vi "read_write_p.vi"() -> ()   [LabVIEW 2020]
uses:
  dxl_x86_c.lvlib/dxl_x86_c.lvlib
panel:
  out "dynamixel_comm_result":string
  out "dynamixel_error":string
  in  "Serial Port":string="COM1"
  in  "ADDR_PRESENT_POSITION":u16=580
  in  "ADDR_GOAL_POSITION":u16=564
  in  "ADDR_TORQUE_ENABLE":u16=512
  out "Protocol Version":dbl=2.0
  out "Present Position":i32(knob) scale=200000.0..-200000.0
  in  "terminate":bool
  out "port_num":i32
  in  "Goal Position":i32(knob) scale=200000.0..-200000.0
  in  "DYNAMIXEL ID":u8=1
  in  "Baud Rate":i32=57600
  # "/*******************************************************************************\n* Copyright (c) 2021, ROBOTIS CO., LTD.\n* All rights reserved.\n*\n* Redistribution and use in source and binary forms, with or without\n* modification, are permitted provided that the following conditions are met:\n*\n* * Redistributions of source code must retain the above copyright notice, this\n*   list of conditions and the following disclaimer.\n*\n* * Redistributions in binary form must reproduce the above copyright notice,\n*   this list of conditions and the following disclaimer in the documentation\n*   and/or other materials provided with the distribution.\n*\n* * Neither the name of ROBOTIS nor the names of its\n*   contributors may be used to endorse or promote products derived from\n*   this software without specific prior written permission.\n*\n* THIS SOFTWARE IS PROVIDED BY THE COPYRIGHT HOLDERS AND CONTRIBUTORS \"AS IS\"\n* AND ANY EXPRESS OR IMPLIED WARRANTIES, INCLUDING, BUT NOT LIMITED TO, THE\n* IMPLIED WARRANTIES OF MERCHANTABILITY AND FITNESS FOR A PARTICULAR PURPOSE ARE\n* DISCLAIMED. IN NO EVENT SHALL THE COPYRIGHT HOLDER OR CONTRIBUTORS BE LIABLE\n* FOR ANY DIRECT, INDIRECT, INCIDENTAL, SPECIAL, EXEMPLARY, OR CONSEQUENTIAL\n* DAMAGES (INCLUDING, BUT NOT LIMITED TO, PROCUREMENT OF SUBSTITUTE GOODS OR\n* SERVICES; LOSS OF USE, DATA, OR PROFITS; OR BUSINESS INTERRUPTION) HOWEVER\n* CAUSED AND ON ANY THEORY OF LIABILITY, WHETHER IN CONTRACT, STRICT LIABILITY,\n* OR TORT (INCLUDING NEGLIGENCE OR OTHERWISE) ARISING IN ANY WAY OUT OF THE USE\n* OF THIS SOFTWARE, EVEN IF ADVISED OF THE POSSIBILITY OF SUCH DAMAGE.\n*******************************************************************************/\n\n/* Author: Ryu Woon Jung (Leon), Will Son */"
  # "[How to run the example]\n1. Connect the U2D2 and DYNAMIXEL to the PC\n2. Confirm the Serial Port number that is assigned to the U2D2 from the Device Manager.\n3. Click the \"Run\" button to run the example.\n4. Drag the Goal Position dial knob or enter the value in the textbox underneath\n5. To finish the example, press \"Quit\" button. (Quitting with \"Abort Execution\" may cause port issue)\n\nSupported DYNAMIXEL with this example :\n  - All P series\n  - PRO(A) series : PRO series with Advanced firmware\n  - PRO series requires modification in ADDR_* fields\n\nThis example is designed for running DYNAMIXEL with U2D2.\nOther DYNAMIXEL such as X or PRO series can be run by modifying below address based on eManual.\nhttps://emanual.robotis.com\n  - ADDR_TORQUE_ENABLE\n  - ADDR_GOAL_POSITION\n  - ADDR_PRESENT_POSITION\n\nMake sure that your DYNAMIXEL is set to ID = 1, Baud Rate = 57600\nThese are the factory default setting of P series\n\nPlease note each P series have different MIN / MAX Position limits."
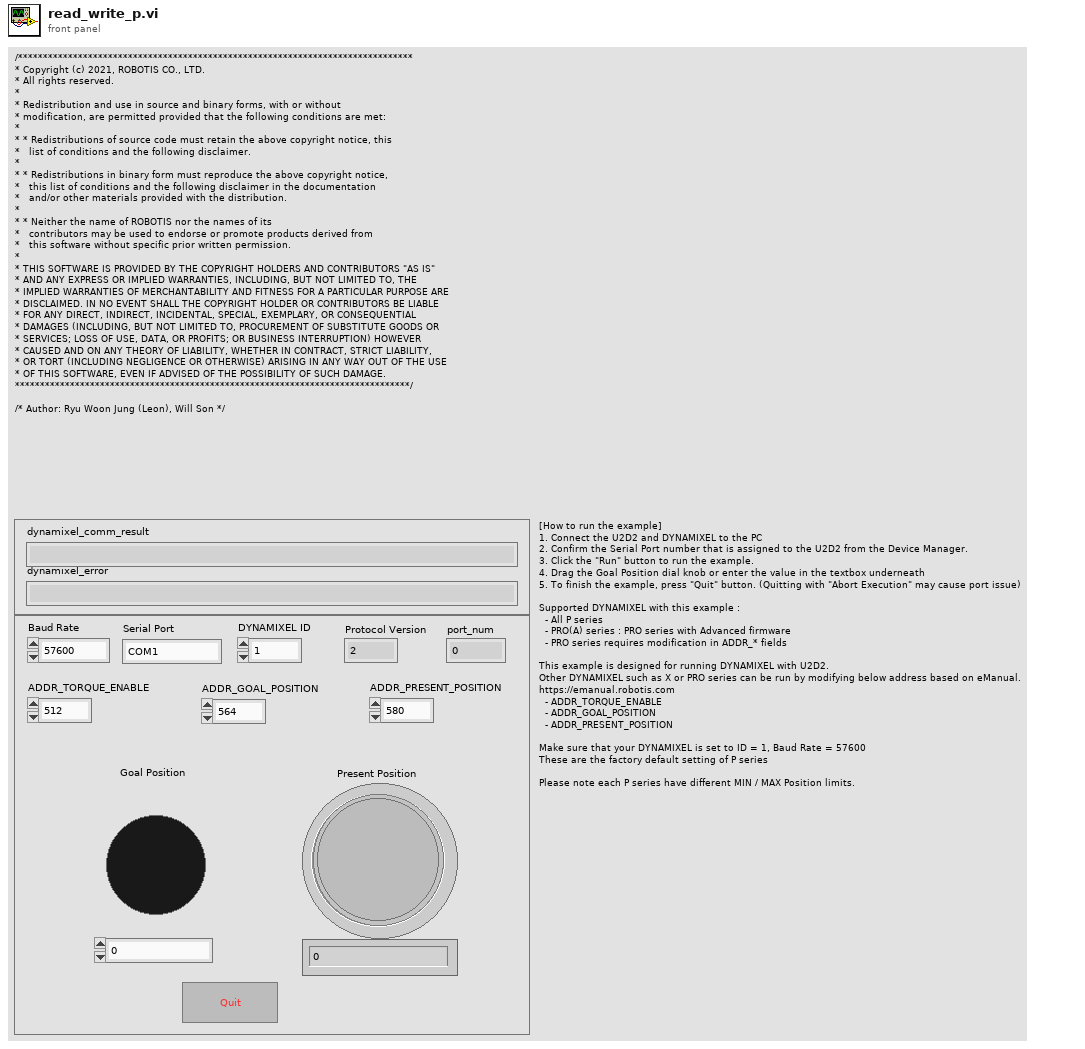
[diagram p1: front panel]
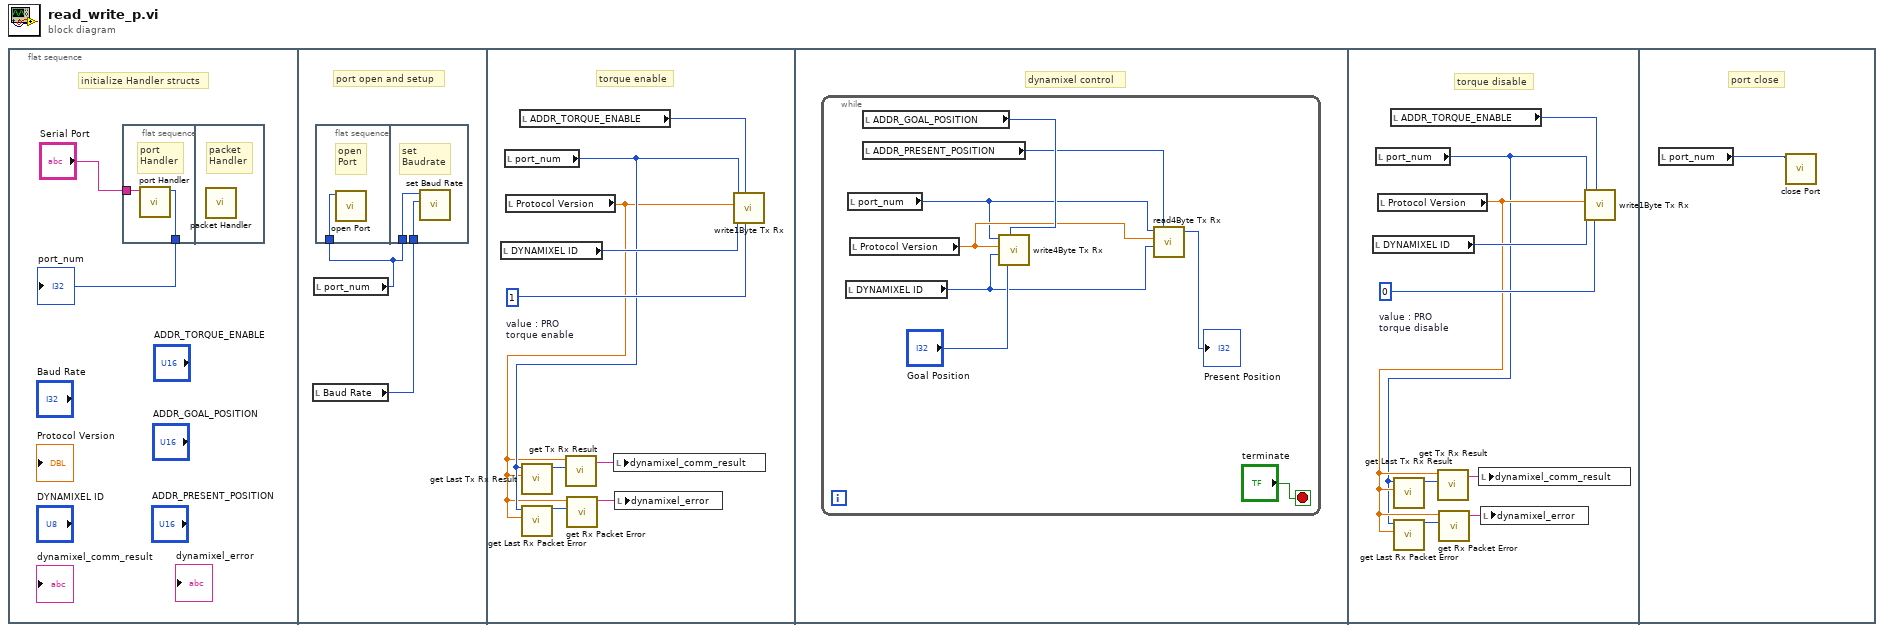
[diagram p0: block diagram]
diagram:
  n1 = flat-sequence {
    frame #0 {
      # "initialize Handler structs"
      n2 = flat-sequence {
        tunnel: [w4] -> w2
        tunnel: "Serial Port" -> [w3]
        frame #0 {
          # "port\nHandler"
          n3 = call "port Handler.vi"("port_name"=w3) -> ("function return"=w4:i32)  [unwired: 10 in]
        }
        frame #1 {
          # "packet\nHandler"
          n4 = call "packet Handler.vi"() -> ()  [unwired: 12 in]
        }
      }
      "port_num" <- w2
    }
    frame #1 {
      # "port open and setup"
      n5 = local read "Baud Rate"() -> (w5:i32)
      n6 = local read "port_num"() -> (w6:i32)
      n7 = flat-sequence {
        tunnel: w6 -> [w7]
        tunnel: w6 -> [w9]
        tunnel: w5 -> [w8]
        frame #0 {
          # "open\nPort"
          n8 = call "open Port.vi"("port_num"=w7) -> ()  [unwired: 10 in, 1 out]
        }
        frame #1 {
          # "set\nBaudrate"
          n9 = call "set Baud Rate.vi"("baudrate"=w8, "port_num"=w9) -> ()  [unwired: 9 in, 1 out]
        }
      }
    }
    frame #2 {
      w18 = 1  # value : PRO torque enable
      # "torque enable"
      n10 = local read "DYNAMIXEL ID"() -> (w17:u8)
      n11 = local read "port_num"() -> (w13:i32)
      n12 = local read "Protocol Version"() -> (w12:dbl)
      n13 = local read "ADDR_TORQUE_ENABLE"() -> (w16:u16)
      n14 = call "get Last Tx Rx Result.vi"("protocol_version"=w12, "port_num"=w13) -> ("function return"=w15:i32)  [unwired: 9 in]
      n15 = call "get Last Rx Packet Error.vi"("protocol_version"=w12, "port_num"=w13) -> ("function return"=w14:u8)  [unwired: 9 in]
      n16 = call "get Tx Rx Result.vi"("result"=w15, "protocol_version"=w12) -> ("function return"=w10:string)  [unwired: 9 in]
      n17 = call "get Rx Packet Error.vi"("error"=w14, "protocol_version"=w12) -> ("function return"=w11:string)  [unwired: 9 in]
      n18 = local write "dynamixel_comm_result"(w10) -> ()
      n19 = local write "dynamixel_error"(w11) -> ()
      n20 = call "write1Byte Tx Rx.vi"("data"=w18, "address"=w16, "id"=w17, "protocol_version"=w12, "port_num"=w13) -> ()  [unwired: 7 in]
    }
    frame #3 {
      # "dynamixel control"
      n21 = while {
        stop <- "terminate" stop-if-true
        n22 = local read "DYNAMIXEL ID"() -> (w23:u8)
        n23 = local read "port_num"() -> (w21:i32)
        n24 = local read "Protocol Version"() -> (w22:dbl)
        n25 = local read "ADDR_GOAL_POSITION"() -> (w25:u16)
        n26 = local read "ADDR_PRESENT_POSITION"() -> (w20:u16)
        n27 = call "write4Byte Tx Rx.vi"("data"="Goal Position", "address"=w25, "id"=w23, "protocol_version"=w22, "port_num"=w21) -> ()  [unwired: 7 in]
        n28 = call "read4Byte Tx Rx.vi"("address"=w20, "id"=w23, "protocol_version"=w22, "port_num"=w21) -> ("function return"=→"Present Position":u32)  [unwired: 7 in]
      }
    }
    frame #4 {
      w34 = 0  # value : PRO torque disable
      # "torque disable"
      n29 = local read "DYNAMIXEL ID"() -> (w35:u8)
      n30 = local read "port_num"() -> (w29:i32)
      n31 = local read "Protocol Version"() -> (w30:dbl)
      n32 = local read "ADDR_TORQUE_ENABLE"() -> (w33:u16)
      n33 = call "get Last Tx Rx Result.vi"("protocol_version"=w30, "port_num"=w29) -> ("function return"=w31:i32)  [unwired: 9 in]
      n34 = call "get Last Rx Packet Error.vi"("protocol_version"=w30, "port_num"=w29) -> ("function return"=w32:u8)  [unwired: 9 in]
      n35 = call "get Tx Rx Result.vi"("result"=w31, "protocol_version"=w30) -> ("function return"=w28:string)  [unwired: 9 in]
      n36 = call "get Rx Packet Error.vi"("error"=w32, "protocol_version"=w30) -> ("function return"=w27:string)  [unwired: 9 in]
      n37 = local write "dynamixel_comm_result"(w28) -> ()
      n38 = local write "dynamixel_error"(w27) -> ()
      n39 = call "write1Byte Tx Rx.vi"("data"=w34, "address"=w33, "id"=w35, "protocol_version"=w30, "port_num"=w29) -> ()  [unwired: 7 in]
    }
    frame #5 {
      # "port close"
      n40 = local read "port_num"() -> (w36:i32)
      n41 = call "close Port.vi"("port_num"=w36) -> ()  [unwired: 11 in]
    }
  }
